vi "generate_LED_configuration.vi"(4 "error in":errorcluster) -> (0 "error out":errorcluster)   [LabVIEW 2019]
doc: "Generates a JSON string to configure a LED array."
uses:
  controls/LightsConfig.ctl
  controls/lights.ctl
panel:
  in  "Tab Control":T1(tab)
  out "LED Config JSON":string
  out "Lights Configuration":T2
  in  "actor_id":string
  in  "location":cluster{"x":dbl, "y":dbl, "z":dbl}={"x"=171.0, "y"=-54.0, "z"=81.0}
  in  "Initial Yaw offset":dbl=6.0
  in  "array_id":string="LF"
  in  "Number of Lights":i32=8
  out "Current Size":i32
  in  "Y offset":dbl=-2.0
  in  "Yaw offset":dbl=-3.0
  in  "Button 1":bool
  in  "stop":bool
  # "RF"
  # "Initial Yaw offset = -6"
  # "Y offset = 2"
  # "Yaw offset = 3"
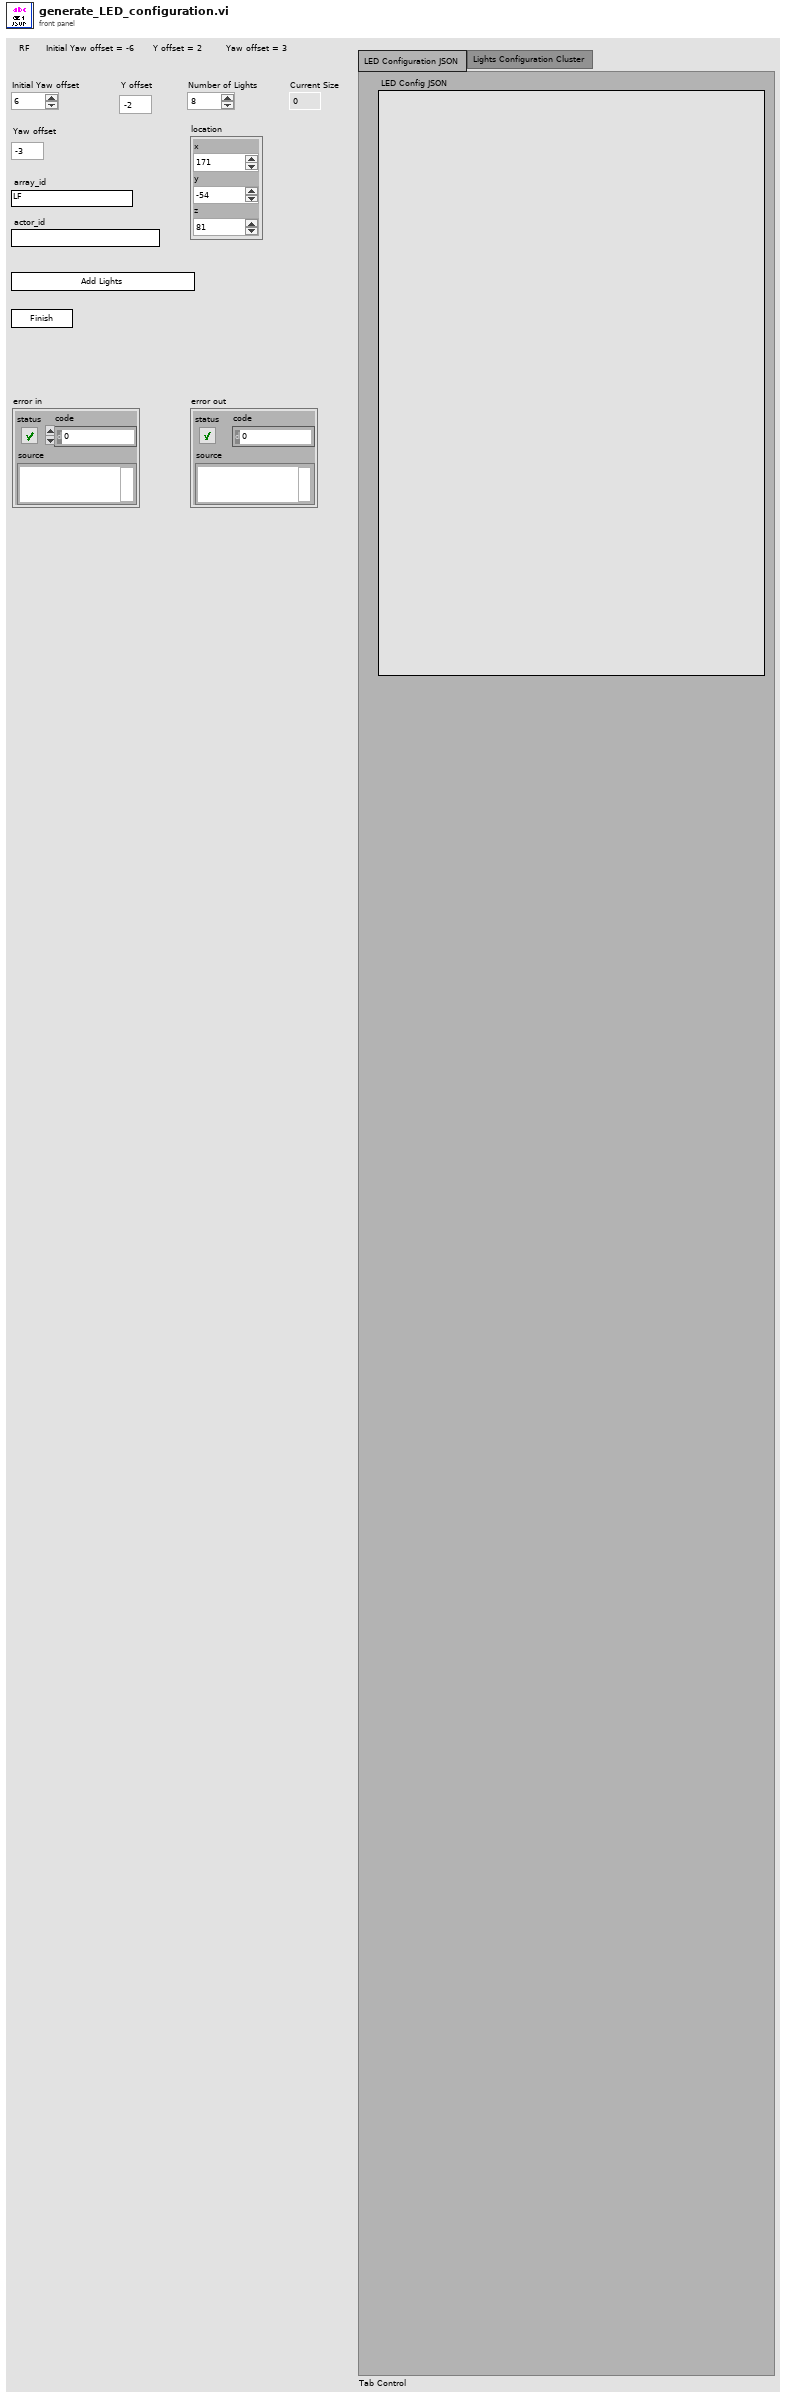
[diagram p1: front panel]
types:
  T1 = enum32{"LED Configuration JSON", "Lights Configuration Cluster"}
  T2 = typedef "LightsConfig.ctl" = cluster{"actor_id":string, "description":string, "enable_streaming":bool, "lights":cluster{"array_id":string, "description":string, "listen_port":i32, "location":cluster{"x":dbl, "y":dbl, "z":dbl}, "rotation":cluster{"pitch":dbl, "roll":dbl, "yaw":dbl}, "type":string, "lights":T3}[]}
  T3 = typedef "lights.ctl" = cluster{"attenuation_radius":dbl, "backlight_attenuation_radius":dbl, "backlight_color":cluster{"a":i32, "b":i32, "g":i32, "r":i32}, "backlight_indirect_lighting_intensity":dbl, "backlight_intensity":dbl, "backlight_soft_source_radius":dbl, "backlight_source_length":dbl, "backlight_source_radius":dbl, "backlight_temperature":dbl, "backlight_volumetric_scattering_intensity":dbl, "color":cluster{"a":i32, "b":i32, "g":i32, "r":i32}, "ies_profile":string, "indirect_lighting_intensity":dbl, "inner_cone_angle":dbl, "intensity":dbl, "led":i32, "listen_port":i32, "location":cluster{"x":dbl, "y":dbl, "z":dbl}, "outer_cone_angle":dbl, "rotation":cluster{"pitch":dbl, "roll":dbl, "yaw":dbl}, "soft_source_radius":dbl, "source_length":dbl, "source_radius":dbl, "temperature":dbl, "type":string, "volumetric_scattering_intensity":dbl}[]
  T4 = cluster{"array_id":string, "description":string, "listen_port":i32, "location":cluster{"x":dbl, "y":dbl, "z":dbl}, "rotation":cluster{"pitch":dbl, "roll":dbl, "yaw":dbl}, "type":string, "lights":T3}
  T5 = cluster{"attenuation_radius":dbl, "backlight_attenuation_radius":dbl, "backlight_color":cluster{"a":i32, "b":i32, "g":i32, "r":i32}, "backlight_indirect_lighting_intensity":dbl, "backlight_intensity":dbl, "backlight_soft_source_radius":dbl, "backlight_source_length":dbl, "backlight_source_radius":dbl, "backlight_temperature":dbl, "backlight_volumetric_scattering_intensity":dbl, "color":cluster{"a":i32, "b":i32, "g":i32, "r":i32}, "ies_profile":string, "indirect_lighting_intensity":dbl, "inner_cone_angle":dbl, "intensity":dbl, "led":i32, "listen_port":i32, "location":cluster{"x":dbl, "y":dbl, "z":dbl}, "outer_cone_angle":dbl, "rotation":cluster{"pitch":dbl, "roll":dbl, "yaw":dbl}, "soft_source_radius":dbl, "source_length":dbl, "source_radius":dbl, "temperature":dbl, "type":string, "volumetric_scattering_intensity":dbl}
  T6 = cluster{"array_id":string, "description":string, "listen_port":i32, "location":cluster{"x":dbl, "y":dbl, "z":dbl}, "rotation":cluster{"pitch":dbl, "roll":dbl, "yaw":dbl}, "type":string, "lights":T3}[]
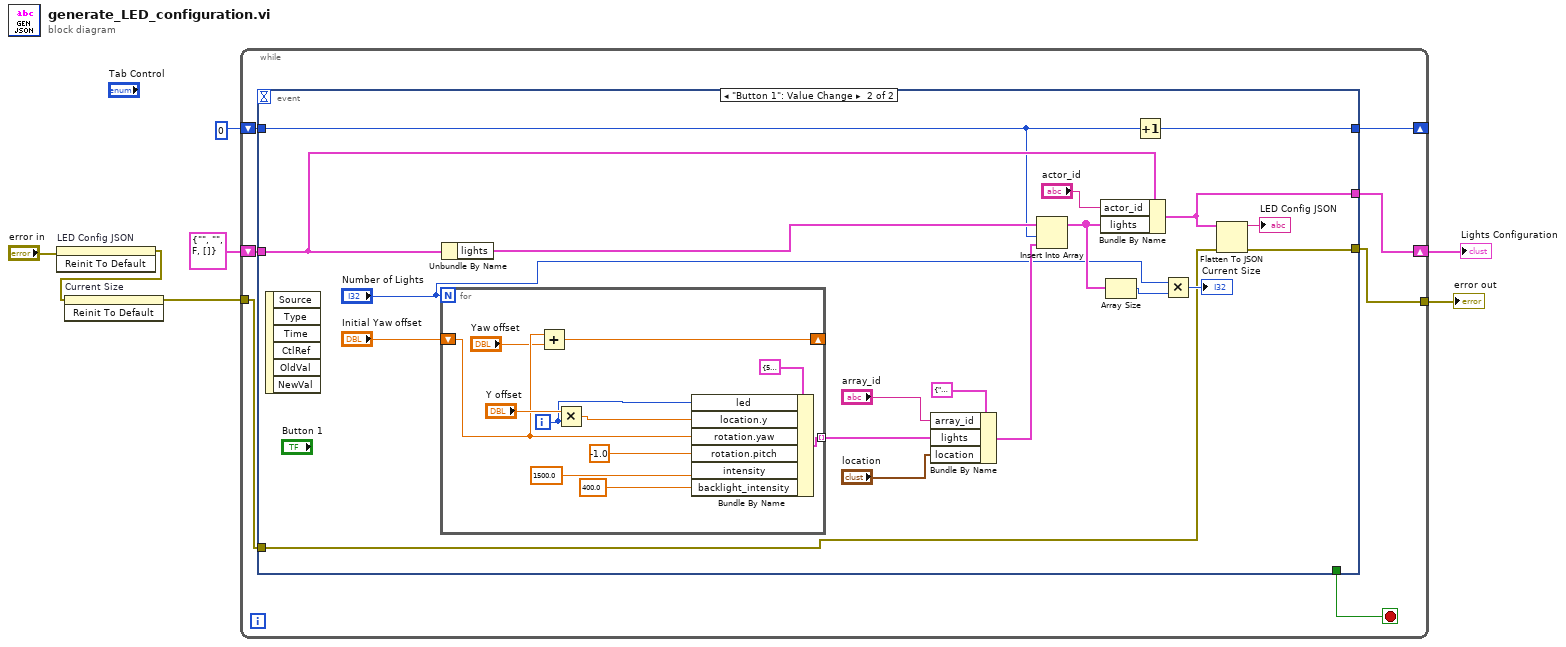
[diagram p0: block diagram]
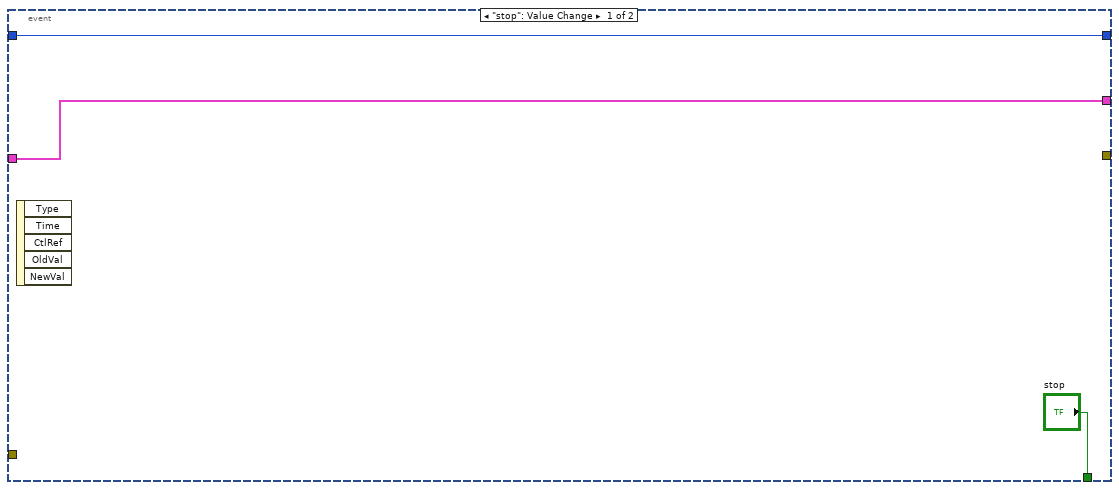
[diagram p2: hidden frame]
diagram:
  n1 = invoke on="LED Config JSON" class="Str" method="Reinit To Default"(error in="error in") -> (error out=w4:errorcluster)  [unwired: 2 in, 2 out]
  n2 = invoke on="Current Size" class="DigNum (strict)" method="Reinit To Default"(error in=w4) -> (error out=w3:errorcluster)  [unwired: 2 in, 2 out]
  n3 = while {
    shift-right: [w12] -> w5
    shift-left: T2 {"actor_id"="", "description"="", "enable_streaming"=FALSE, "lights"=[]} ("LightsConfig") -> [w13]
    shift-right: [w10] -> _
    shift-left: 0 -> [w11]
    tunnel: w3 -> [w9]
    tunnel: [w8] -> w1
    stop <- w14 stop-if-true
    n4 = event shown="[1] \"Button 1\": Value Change" {
      selector: _ -> [_ _]
      dyn-events: _ -> [_ _]
      timeout: _ -> [_ _]
      tunnel: ["stop" _] -> w14
      tunnel: w13 -> [w16 w31]
      tunnel: [w16 w27] -> w12
      tunnel: w11 -> [w15 w30]
      tunnel: [w15 w29] -> w10
      tunnel: [_ w20] -> w8
      tunnel: w9 -> [_ w19]
      event "stop": Value Change {
        n5 = event-data() -> ()  [unwired: 1 in, 5 out]
      }
      event "Button 1": Value Change {
        n6 = event-data() -> ()  [unwired: 1 in, 6 out]
        n7 = for {
          N: "Number of Lights" -> [_]
          shift-right: [w43] -> _
          shift-left: "Initial Yaw offset" -> [w45]
          tunnel: [w41] -> w25 mode=indexing
          i -> [w40]
          n8 = Add(x=w45, y="Yaw offset") -> (x+y=w43:dbl)
          n9 = Multiply(x="Y offset", y=w40) -> (x*y=w47:dbl)
          n10 = Bundle By Name(cluster=T5 {"attenuation_radius"=5000.0, "backlight_attenuation_radius"=10.0, "backlight_color"={"a"=255, "b"=255, "g"=255, "r"=255}, "backlight_indirect_lighting_intensity"=10.0, "backlight_intensity"=400.0, "backlight_soft_source_radius"=2.0, "backlight_source_length"=1.0, "backlight_source_radius"=1.0, "backlight_temperature"=8000.0, "backlight_volumetric_scattering_intensity"=10.0, "color"={"a"=255, "b"=255, "g"=255, "r"=255}, "ies_profile"="", "indirect_lighting_intensity"=1.0, "inner_cone_angle"=2.0, "intensity"=1500.0, "led"=0, "listen_port"=0, "location"={"x"=0.0, "y"=0.0, "z"=0.0}, "outer_cone_angle"=6.0, "rotation"={"pitch"=0.0, "roll"=0.0, "yaw"=0.0}, "soft_source_radius"=0.0, "source_length"=1.0, "source_radius"=0.0, "temperature"=8000.0, "type"="", "volumetric_scattering_intensity"=5.0}, "led"=w40, "location.y"=w47, "rotation.yaw"=w45, "rotation.pitch"=-1.0, "intensity"=1500.0, "backlight_intensity"=400.0) -> (w41:T5)
        }
        n11 = Unbundle By Name(w31) -> ("lights"=w32:T6)
        n12 = Bundle By Name(cluster=T4 {"array_id"="", "description"="", "listen_port"=0, "location"={"x"=0.0, "y"=0.0, "z"=0.0}, "rotation"={"pitch"=0.0, "roll"=0.0, "yaw"=0.0}, "type"="", "lights"=[]} ("new element/subarray"), "array_id"="array_id", "lights"=w25, "location"="location") -> (w24:T4)
        n13 = Insert Into Array(array=w32, index=w30, new element=w24) -> (w36:T6)
        n14 = Bundle By Name(cluster=w31, "actor_id"="actor_id", "lights"=w36) -> (w27:T2)
        n15 = Array Size(array=w36) -> (size(s)=w35:i32)
        n16 = Increment(x=w30) -> (x+1=w29:i32)
        n17 = Multiply(x="Number of Lights", y=w35) -> (x*y=→"Current Size":i32)
        n18 = Flatten To JSON(anything=w27, error in (no error)=w19) -> (JSON string=→"LED Config JSON":string, 11:w20:errorcluster)  [unwired: 1 in]
      }
    }
  }
  "Lights Configuration" <- w5
  "error out" <- w1
